vi "Keithley K2400 Address constant.vi"() -> ()   [LabVIEW 2020]
panel:
  in  "Keithley K2400 Address":string="24"
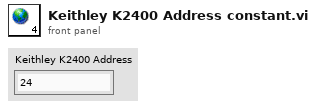
[diagram p1: front panel]
diagram:
